vi "wait4trig.vi"(8 "error in":errorcluster, 11 "task/channels in":refnum<k21>) -> (0 "error out":errorcluster, 2 "voltage out":dbl, 3 "task out":refnum<k21>)   [LabVIEW 2015]
uses:
  <vilib>/DAQmx/read.llb/DAQmx Read (Analog DBL 1Chan 1Samp).vi
  <vilib>/DAQmx/miscellaneous.llb/DAQmx Fill In Error Info.vi
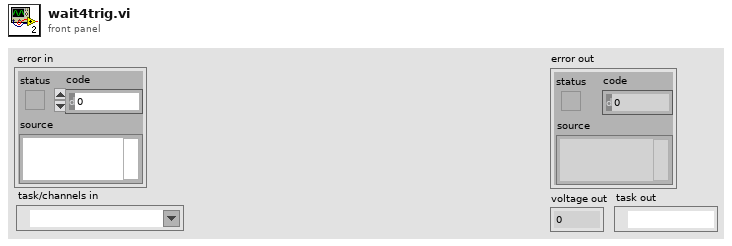
[diagram p1: front panel]
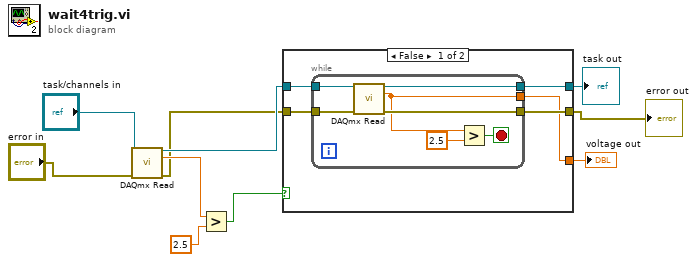
[diagram p0: block diagram]
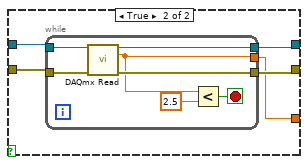
[diagram p2: hidden frame]
diagram:
  n1 = call-poly <vilib>:"DAQmx Read.vi"("task/channels in"="task/channels in", "error in"="error in") -> ("task out"=w7:refnum<k21>, "data"=w10:dbl, "error out"=w6:errorcluster)  [unwired: 11 in]
  n2 = Greater?(x=w10, y=2.5) -> (0:w8:bool)
  n3 = case shown="False" w8 {
    tunnel: [w15 w25] -> w1
    tunnel: [w14 w24] -> w3
    tunnel: w7 -> [w13 w27]
    tunnel: w6 -> [w12 w26]
    tunnel: [w11 w23] -> w5
    frame False {
      n4 = while {
        tunnel: w13 -> [w22]
        tunnel: w12 -> [w21]
        tunnel: [w18] -> w15
        tunnel: [w17] -> w14
        tunnel: [w16] -> w11
        stop <- w19 stop-if-true
        n5 = call-poly <vilib>:"DAQmx Read.vi"("task/channels in"=w22, "error in"=w21) -> ("task out"=w18:refnum<k21>, "data"=w16:dbl, "error out"=w17:errorcluster)  [unwired: 11 in]
        n6 = Greater?(x=w16, y=2.5) -> (0:w19:bool)
      }
    }
    frame True {
      n7 = while {
        tunnel: w27 -> [w34]
        tunnel: w26 -> [w33]
        tunnel: [w30] -> w25
        tunnel: [w29] -> w24
        tunnel: [w28] -> w23
        stop <- w31 stop-if-true
        n8 = call-poly <vilib>:"DAQmx Read.vi"("task/channels in"=w34, "error in"=w33) -> ("task out"=w30:refnum<k21>, "data"=w28:dbl, "error out"=w29:errorcluster)  [unwired: 11 in]
        n9 = Less?(x=w28, y=2.5) -> (x < y?=w31:bool)
      }
    }
  }
  "error out" <- w3
  "voltage out" <- w5
  "task out" <- w1
